vi "3D Viewer.vi"(6 "Initialize ?":bool, 7 "3D View Image":refnum<vi>, 8 "error in (no error)":errorcluster, 9 "Angle Z":sgl, 10 "Angle Y":sgl, 11 "Angle X":sgl) -> (0 "error out":errorcluster, 3 "3D View Image (Local)":refnum<vi>(3d-picture))   [LabVIEW 2017]
uses:
  <vilib>/picture/3D Picture Control/Object/Create Object (drawable).vi
  <vilib>/picture/3D Picture Control/Object/Add Object (no reference).vi
  <vilib>/picture/3D Picture Control/NI_3D Picture Control.lvlib
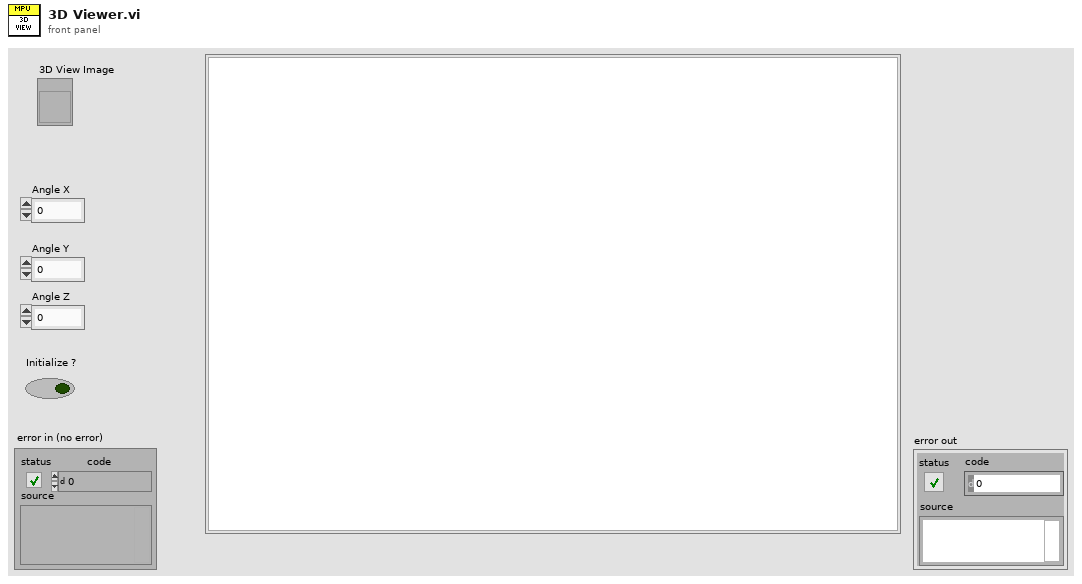
[diagram p1: front panel]
types:
  T1 = cluster{"Red":sgl, "Green":sgl, "Blue":sgl, "Alpha":sgl}
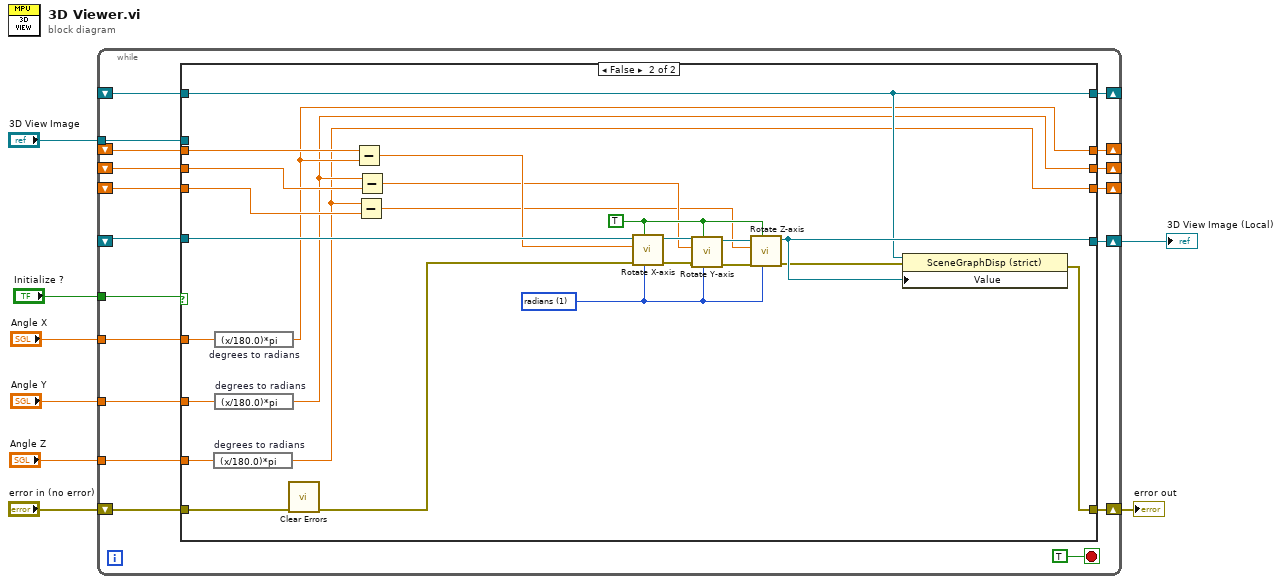
[diagram p0: block diagram]
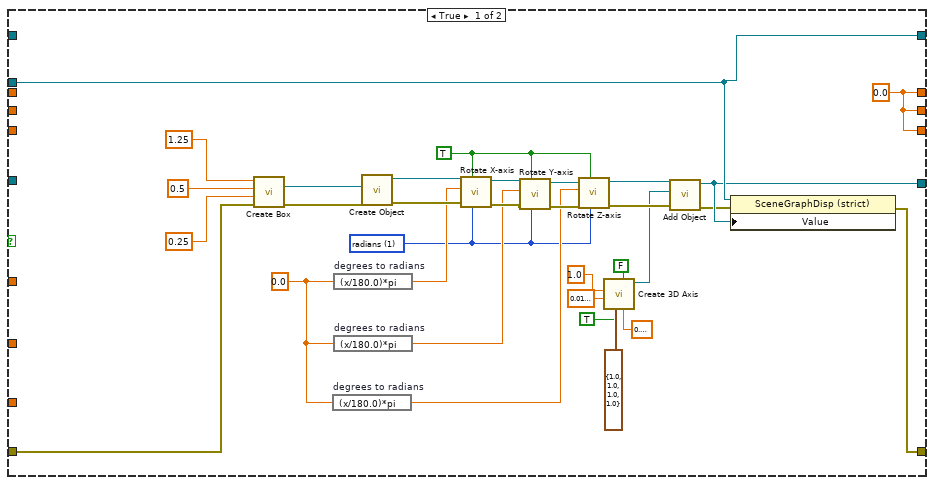
[diagram p2: hidden frame]
diagram:
  n1 = while {
    tunnel: "Angle X" -> [w26]
    tunnel: "Angle Y" -> [w25]
    tunnel: "Angle Z" -> [w24]
    tunnel: "3D View Image" -> [w21]
    shift-right: [w20] -> _
    shift-left: _ -> [w16]
    shift-right: [w23] -> w5
    shift-left: _ -> [w15]
    tunnel: "Initialize ?" -> [w19]
    shift-right: [w17] -> w1
    shift-left: "error in (no error)" -> [w18]
    shift-right: [w14] -> _
    shift-left: _ -> [w11]
    shift-right: [w13] -> _
    shift-left: _ -> [w10]
    shift-right: [w12] -> _
    shift-left: _ -> [w9]
    stop <- TRUE stop-if-true
    n2 = case shown="False" w19 {
      tunnel: w26 -> [_ w83]
      tunnel: w25 -> [_ w80]
      tunnel: w24 -> [_ w77]
      tunnel: [w33 w74] -> w23
      tunnel: w21 -> [w34 _]
      tunnel: [w34 w70] -> w20
      tunnel: w18 -> [w30 w71]
      tunnel: [w29 w72] -> w17
      tunnel: w16 -> [_ w70]
      tunnel: w15 -> [_ w69]
      tunnel: [w27 w64] -> w14
      tunnel: [w27 w63] -> w13
      tunnel: [w27 w62] -> w12
      tunnel: w11 -> [_ w67]
      tunnel: w10 -> [_ w66]
      tunnel: w9 -> [_ w65]
      frame True {
        w27 = 0.0
        w28 = sgl 0.0 ("Angle X")
        w44 = TRUE ("Relative?")
        w45 = u16 1 items=["degree", "radians"] ("angle unit")
        n3 = call <vilib>:"Create Box.vi"("error in (no error)"=w30, "Length Z"=sgl 0.25, "Length Y"=sgl 0.5, "Length X"=sgl 1.25) -> ("error out"=w31:errorcluster, "New Box Refnum"=w58:refnum<vi>)  [unwired: 6 in]
        n4 = expression code="(x/180.0)*pi" "degrees to radians"(w28) -> (w46:sgl)
        n5 = expression code="(x/180.0)*pi" "degrees to radians"(w28) -> (w52:sgl)
        n6 = expression code="(x/180.0)*pi" "degrees to radians"(w28) -> (w49:sgl)
        n7 = call-poly <vilib>:"Create Object.vi"("error in (no error)"=w31, "Geometry"=w58) -> ("error out"=w53:errorcluster, "Scene:New Object"=w54:refnum<vi>)  [unwired: 8 in]
        n8 = call <vilib>:"Rotate X-axis.vi"("angle unit"=w45, "Relative?"=w44, "error in (no error)"=w53, "angle"=w52, "Scene Object In"=w54) -> ("error out"=w50:errorcluster, "Scene Object Out"=w51:refnum<vi>)  [unwired: 5 in]
        n9 = call <vilib>:"Rotate Y-axis.vi"("angle unit"=w45, "Relative?"=w44, "error in (no error)"=w50, "angle"=w49, "Scene Object In"=w51) -> ("error out"=w48:errorcluster, "Scene Object Out"=w47:refnum<vi>)  [unwired: 5 in]
        n10 = call <vilib>:"Rotate Z-axis.vi"("angle unit"=w45, "Relative?"=w44, "error in (no error)"=w48, "angle"=w46, "Scene Object In"=w47) -> ("error out"=w42:errorcluster, "Scene Object Out"=w43:refnum<vi>)  [unwired: 5 in]
        n11 = call <vilib>:"Create 3D Axis.vi"("Character Size"=sgl 0.1, "Half plane?"=FALSE, "Axis label?"=TRUE, "Color"=T1 {"Red"=1.0, "Green"=1.0, "Blue"=1.0, "Alpha"=1.0}, "Radius"=sgl 0.02, "Length"=sgl 1.0) -> ("New Object Refnum"=w35:refnum<vi>)  [unwired: 4 in, 1 out]
        n12 = call-poly <vilib>:"Add Object.vi"("error in (no error)"=w42, "New Object In"=w35, "Scene Object In"=w43) -> ("error out"=w32:errorcluster, "Scene Object Out"=w33:refnum<vi>)  [unwired: 7 in]
        n13 = property class="SceneGraphDisp (strict)"(reference=w34, error in=w32, "Value"=w33) -> (error out=w29:errorcluster)  [unwired: 1 out]
      }
      frame False {
        w75 = TRUE ("Relative?")
        w76 = u16 1 items=["degree", "radians"] ("angle unit")
        n14 = expression code="(x/180.0)*pi" "degrees to radians"(w77) -> (w62:sgl)
        n15 = expression code="(x/180.0)*pi" "degrees to radians"(w83) -> (w64:sgl)
        n16 = expression code="(x/180.0)*pi" "degrees to radians"(w80) -> (w63:sgl)
        n17 = call <vilib>:"Clear Errors.vi"("error in (no error)"=w71) -> ("error out"=w68:errorcluster)  [unwired: 5 in, 1 out]
        n18 = Subtract(x=w67, y=w64) -> (x-y=w61:dbl)
        n19 = Subtract(x=w62, y=w65) -> (x-y=w59:dbl)
        n20 = Subtract(x=w63, y=w66) -> (x-y=w60:dbl)
        n21 = call <vilib>:"Rotate X-axis.vi"("angle unit"=w76, "Relative?"=w75, "error in (no error)"=w68, "angle"=w61, "Scene Object In"=w69) -> ("error out"=w81:errorcluster, "Scene Object Out"=w82:refnum<vi>)  [unwired: 5 in]
        n22 = call <vilib>:"Rotate Y-axis.vi"("angle unit"=w76, "Relative?"=w75, "error in (no error)"=w81, "angle"=w60, "Scene Object In"=w82) -> ("error out"=w79:errorcluster, "Scene Object Out"=w78:refnum<vi>)  [unwired: 5 in]
        n23 = call <vilib>:"Rotate Z-axis.vi"("angle unit"=w76, "Relative?"=w75, "error in (no error)"=w79, "angle"=w59, "Scene Object In"=w78) -> ("error out"=w73:errorcluster, "Scene Object Out"=w74:refnum<vi>)  [unwired: 5 in]
        n24 = property class="SceneGraphDisp (strict)"(reference=w70, error in=w73, "Value"=w74) -> (error out=w72:errorcluster)  [unwired: 1 out]
      }
    }
  }
  "3D View Image (Local)" <- w5
  "error out" <- w1
